vi "LaserONOFFLDC501.vi"(8 "error in (no error)":errorcluster, 9 "LD Setting Point (If ON)":dbl, 10 "Currnet ON/OFF":bool, 11 "VISA resource name":refnum<visa-resource-name>) -> (0 "error out":errorcluster, 3 "VISA resource name out":refnum<visa-resource-name>)   [LabVIEW 2021]
panel:
  out "F-format string":string
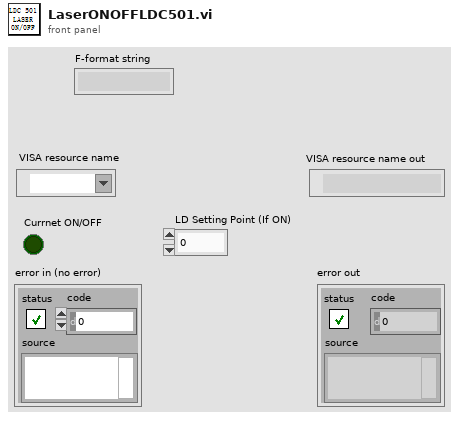
[diagram p1: front panel]
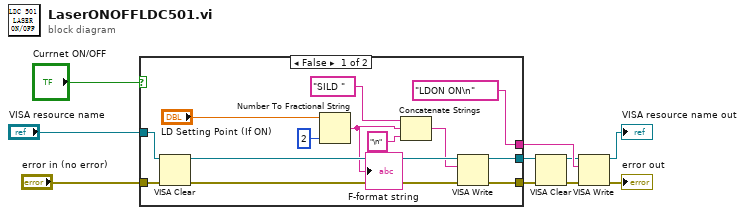
[diagram p0: block diagram]
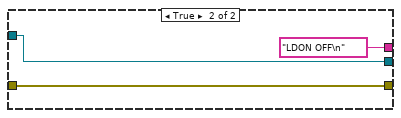
[diagram p2: hidden frame]
diagram:
  n1 = case shown="False" "Currnet ON/OFF" {
    tunnel: ["LDON ON\n" ("write buffer") "LDON OFF\n" ("write buffer")] -> w7
    tunnel: "VISA resource name" -> [w21 w24]
    tunnel: "error in (no error)" -> [w20 w25]
    tunnel: [w19 w25] -> w2
    tunnel: [w18 w24] -> w1
    frame False {
      n2 = VISA Clear(VISA resource name=w21, error in (no error)=w20) -> (VISA resource name out=w17:refnum<visa-resource-name>, error out=w22:errorcluster)
      n3 = Number To Fractional String(number="LD Setting Point (If ON)", precision (6)=i16 2) -> (F-format string=w11:string)  [unwired: 2 in]
      "F-format string" <- w11
      n4 = Concatenate Strings("SILD " ("write buffer"), w11, "\n" ("write buffer")) -> (w14:string)
      n5 = VISA Write(VISA resource name=w17, write buffer=w14, error in (no error)=w22) -> (VISA resource name out=w18:refnum<visa-resource-name>, error out=w19:errorcluster)  [unwired: 1 out]
    }
    frame True {
    }
  }
  n6 = VISA Clear(VISA resource name=w1, error in (no error)=w2) -> (VISA resource name out=w5:refnum<visa-resource-name>, error out=w6:errorcluster)
  n7 = VISA Write(VISA resource name=w5, write buffer=w7, error in (no error)=w6) -> (VISA resource name out=→"VISA resource name out":refnum<visa-resource-name>, error out=→"error out":errorcluster)  [unwired: 1 out]
